vi "SMTP Email Send Data Charset.vi"(0 "recipients":string[](array[string]), 1 "mail server":string, 2 "return address":string, 3 "character set (us-ascii)":string="us-ascii", 5 "subject ([No Subject])":string="[No Subject]", 7 "message":string, 9 "data":string, 11 "error in (no error)":errorcluster, 12 "binary? (F)":bool, 13 "MIME content-type (application/octet-stream)":string="application/octet-stream", 14 "translit":string="MacRoman iso-8859-1 macroman.trl, ToUpper iso-8859-1 toupper.trl,\nMacRomanUp MacRoman toupper.trl") -> (4 "invalid recipients":string[](array[string]), 15 "error out":errorcluster)   [LabVIEW 2009, in "NewNI_SMTPEmail.lvlib"]
doc: "Sends an email with attached data to a list of recipients."
uses:
  NewNI_SMTPEmail.lvlib
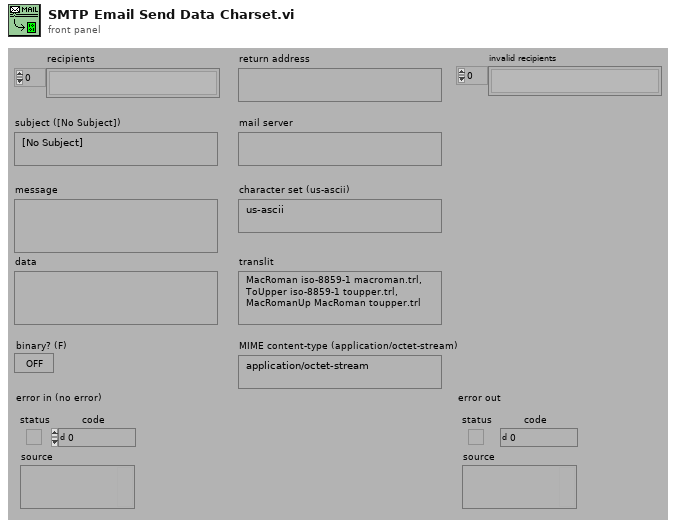
[diagram p1: front panel]
types:
  T1 = cluster{path, "data":string, "binary? (F)":bool, "MIME content-type (application/octet-stream)":string}
  T2 = typedef "NewNI_SMTPEmail.lvlib/SMTP Email Session.ctl" = refnum<k1>
  T3 = cluster{path, "data":string, "binary? (F)":bool, "MIME content-type (application/octet-stream)":string}[]
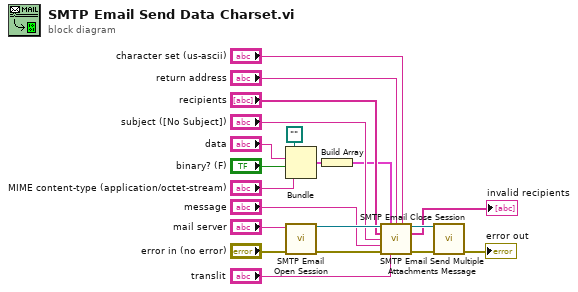
[diagram p0: block diagram]
diagram:
  n1 = Bundle(path "", "data"="data", "binary? (F)"="binary? (F)", "MIME content-type (application/octet-stream)"="MIME content-type (application/octet-stream)") -> (w17:T1)  [unwired: 1 out]
  n2 = call "SMTP Email Open Session.vi"("error in (no error)"="error in (no error)", "mail server"="mail server") -> ("error out"=w15:errorcluster, "smtp session out"=w14:T2)  [unwired: 1 in, 3 out]
  n3 = Build Array(w17) -> (w3:T3)
  n4 = call "SMTP Email Send Multiple Attachments Message.vi"("smtp session"=w14, "attachments"=w3, "return address"="return address", "character set"="character set (us-ascii)", "recipients"="recipients", "subject"="subject ([No Subject])", "message"="message", "error in (no error)"=w15, "translit"="translit") -> ("smtp session out"=w13:T2, "invalid recipients"=→"invalid recipients":string[], "error out"=w12:errorcluster)  [unwired: 4 out]
  n5 = call "SMTP Email Close Session.vi"("error in (no error)"=w12, "smtp session"=w13) -> ("error out"=→"error out":errorcluster)  [unwired: 5 out]
